vi "Sand Fall.vi"(6 "Next Location":cdb, 7 "Rock Grid":set{cdb}(c389), 8 "Current Location in":cdb, 9 "Bounds":T1, 11 "Sand Grid in":set{cdb}(c389)) -> (0 "Current Location out":cdb, 1 "Sand Reached Resting Position ?":bool, 3 "Sand Grid out":set{cdb}(c389), 4 "Arrived at Decision ?":bool, 5 "Falling into Void ?":bool)   [LabVIEW 2020, in "AoC 2022.lvlib"]
uses:
  AoC 2022.lvlib
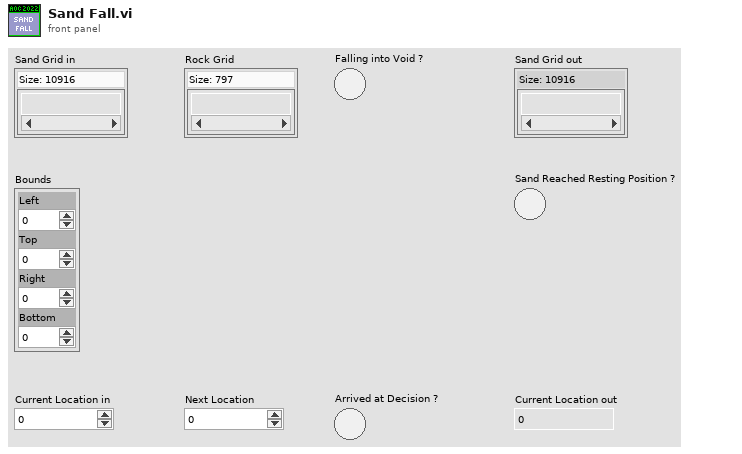
[diagram p1: front panel]
types:
  T1 = cluster{"Left":i16, "Top":i16, "Right":i16, "Bottom":i16}
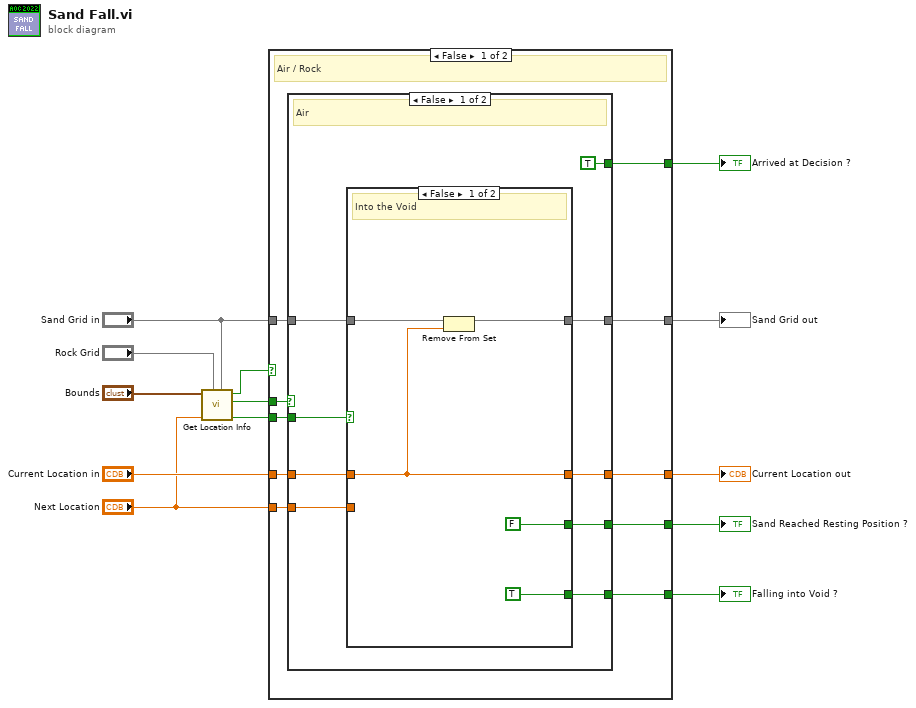
[diagram p0: block diagram]
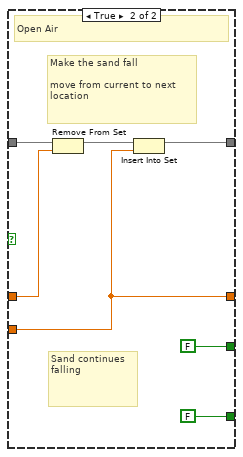
[diagram p2: hidden frame]
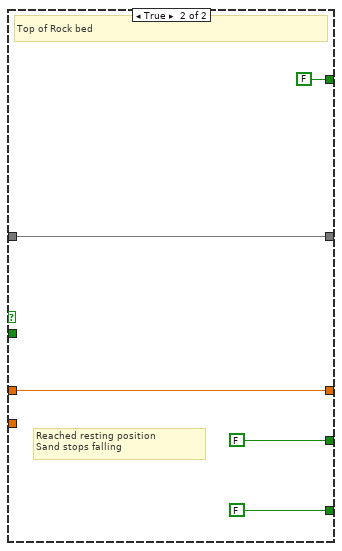
[diagram p3: hidden frame]
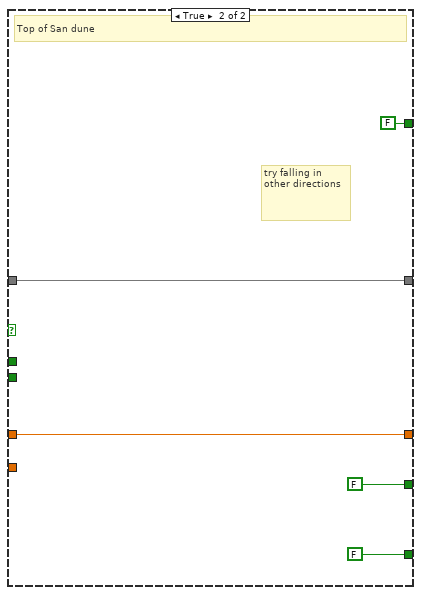
[diagram p4: hidden frame]
diagram:
  n1 = call "Get Location Info.vi"("Sand Grid"="Sand Grid in", "Rock Grid"="Rock Grid", "Location"="Next Location", "Grid Bounds"="Bounds") -> ("Within the Grid ?"=w11:bool, "Filled with Rock ?"=w6:bool, "Filled with Sand ?"=w12:bool)  [unwired: 3 in]
  n2 = case shown="False" w12 {
    tunnel: "Sand Grid in" -> [w23 w54]
    tunnel: w6 -> [w22 _]
    tunnel: [w21 FALSE] -> w7
    tunnel: [w20 w54] -> w8
    tunnel: [w19 FALSE] -> w9
    tunnel: [w18 w53] -> w10
    tunnel: "Next Location" -> [w17 _]
    tunnel: w11 -> [w16 _]
    tunnel: "Current Location in" -> [w15 w53]
    tunnel: [w14 FALSE] -> w13
    frame False {
      # "Air / Rock"
      n3 = case shown="False" w22 {
        tunnel: [w28 FALSE] -> w21
        tunnel: [w27 FALSE] -> w19
        tunnel: [w31 w47] -> w20
        tunnel: w23 -> [w30 w47]
        tunnel: w17 -> [w26 _]
        tunnel: [w29 w46] -> w18
        tunnel: w16 -> [w32 _]
        tunnel: w15 -> [w25 w46]
        tunnel: [TRUE FALSE] -> w14
        frame False {
          # "Air"
          n4 = case shown="False" w32 {
            tunnel: [w34 w42] -> w31
            tunnel: w30 -> [w35 w40]
            tunnel: [w33 w41] -> w29
            tunnel: [FALSE FALSE] -> w28
            tunnel: [TRUE FALSE] -> w27
            tunnel: w26 -> [_ w41]
            tunnel: w25 -> [w33 w38]
            frame False {
              # "Into the Void"
              n5 = Remove From Set(10:w33, 11:w35) -> (3:w34:set{cdb})  [unwired: 1 out]
            }
            frame True {
              # "Make the sand fall\n\nmove from current to next location"
              # "Sand continues falling"
              # "Open Air"
              n6 = Remove From Set(10:w38, 11:w40) -> (3:w39:set{cdb})  [unwired: 1 out]
              n7 = Insert Into Set(10:w41, 11:w39) -> (3:w42:set{cdb})  [unwired: 1 out]
            }
          }
        }
        frame True {
          # "Reached resting position\nSand stops falling"
          # "Top of Rock bed"
        }
      }
    }
    frame True {
      # "try falling in other directions"
      # "Top of San dune"
    }
  }
  "Arrived at Decision ?" <- w13
  "Current Location out" <- w10
  "Falling into Void ?" <- w9
  "Sand Grid out" <- w8
  "Sand Reached Resting Position ?" <- w7
